vi "未命名 5.vi"(0 "Image In":T3, 1 "Image Dst":T3, 2 "ROI Descriptor (Pattern Matching 1)":T2={"Global Rectangle"=[20, 78, 890, 919], "Contours"=[{"ID"=enum."External", "Type"=12, "Coordinates"=[20, 78, 890, 919, 0]}]} {"Contours"."Type" items=["No Selection", "Point", "Line", "Rectangle", "Oval", "Polygon", "Freehand Region", "Annulus", "Unused2", "Unused3", "Broken Line", "Freehand Line", "Rotated Rectangle"]}, 3 "Algorithm (Pattern Matching 1)":i32(ring)=2 items=["All", "Low Discrepancy Sampling", "Grayscale Value Pyramid", "Gradients Pyramid"], 4 "Parameters (Pattern Matching 1)":T1={"Number of Matches Requested"=1, "Minimum Match Score"=800.0, "Angle Ranges"=[]}, 5 "Advanced Options (Pattern Matching 1)":cluster{"Item":u16, "Value":dbl}[](array[cluster])=[{"Item"=102, "Value"=10.0}, {"Item"=106, "Value"=300.0}, {"Item"=107, "Value"=0.0}, {"Item"=108, "Value"=6.0}, {"Item"=109, "Value"=1.0}, {"Item"=114, "Value"=25.0}, {"Item"=111, "Value"=20.0}, {"Item"=112, "Value"=10.0}, {"Item"=113, "Value"=20.0}, {"Item"=103, "Value"=1.0}, {"Item"=104, "Value"=20.0}, {"Item"=105, "Value"=0.0}, {"Item"=100, "Value"=6.0}] {"Item" items=["LD Sampling - Minimum Constrast"=0, "LD Sampling - Enable Subpixel Accuracy"=1, "LD Sampling - Search Strategy"=2, "LD Sampling - Subpixel Iterations"=3, "LD Sampling - Subpixel Tolerance"=4, "LD Sampling - Initial Match List Length"=5, "LD Sampling - Match List Reduction Factor"=6, "LD Sampling - Initial Step Size"=7, "LD Sampling - Intermediate Angular Accuracy"=8, "-"=9, "Pyramid - Max Pyramid Level"=100, "Pyramid - Minimum Contrast"=102, "Pyramid - Enable Subpixel Accuracy"=103, "Pyramid - Subpixel Iterations"=104, "Pyramid - Subpixel Tolerance"=105, "Pyramid - Initial Match List Length"=106, "Pyramid - Match List Reduction Factor"=107, "Pyramid - Intermediate Angular Accuracy"=108, "Pyramid - Process Border Matches"=109, "Pyramid - Min Match Separation Distance"=111, "Pyramid - Min Match Separation Angle"=112, "Pyramid - Max Match Overlap"=113, "Pyramid - Max Cache in MB"=114, "Pyramid - Clear Cache"=115, "-"=116, "Enable Defect Map"=200]}, 6 "Template File Path (Pattern Matching 1)":path=path "D:/Inspect System/Source Code/Template Program/字符检测定位模板.png", 7 "error in":errorcluster) -> (20 "Image Out":T3, 21 "Matches (Pattern Matching 1)":T4(array[cluster]) {"Bounding Box"."y" format="%.2f"; "Bounding Box"."x" format="%.2f"; "Position"."y" format="%.2f"; "Position"."x" format="%.2f"; "Score" format="%.2f"; "Scale" format="%.2f"; "Angle" format="%.2f"}, 22 "Calibrated Matches (Pattern Matching 1)":T4(array[cluster]) {"Bounding Box"."y" format="%.2f"; "Bounding Box"."x" format="%.2f"; "Position"."y" format="%.2f"; "Position"."x" format="%.2f"; "Score" format="%.2f"; "Scale" format="%.2f"; "Angle" format="%.2f"}, 23 "Number of Matches (Pattern Matching 1)":i32, 27 "error out":errorcluster)   [LabVIEW 2017]
doc: "Creates, edits, and runs vision algorithms using NI Vision Assistant.\n\nWhen you place this Express VI on the block diagram, NI Vision Assistant launches. Create an algorithm using the Vision Assistant processing functions. After you create an algorithm, you can select the controls and indicators that you want to be able to programmatically set in LabVIEW. Double-click the Vision Assistant Express VI to edit the algorithm."
uses:
  <vilib>/vision/Image Controls.llb/IMAQ Image.ctl
  <vilib>/vision/Pattern Matching.llb/IMAQ Curve Parameters.ctl
  <vilib>/vision/Pattern Matching.llb/IMAQ Match Range Setting.ctl
  <vilib>/vision/NI_Vision_Development_Module.lvlib
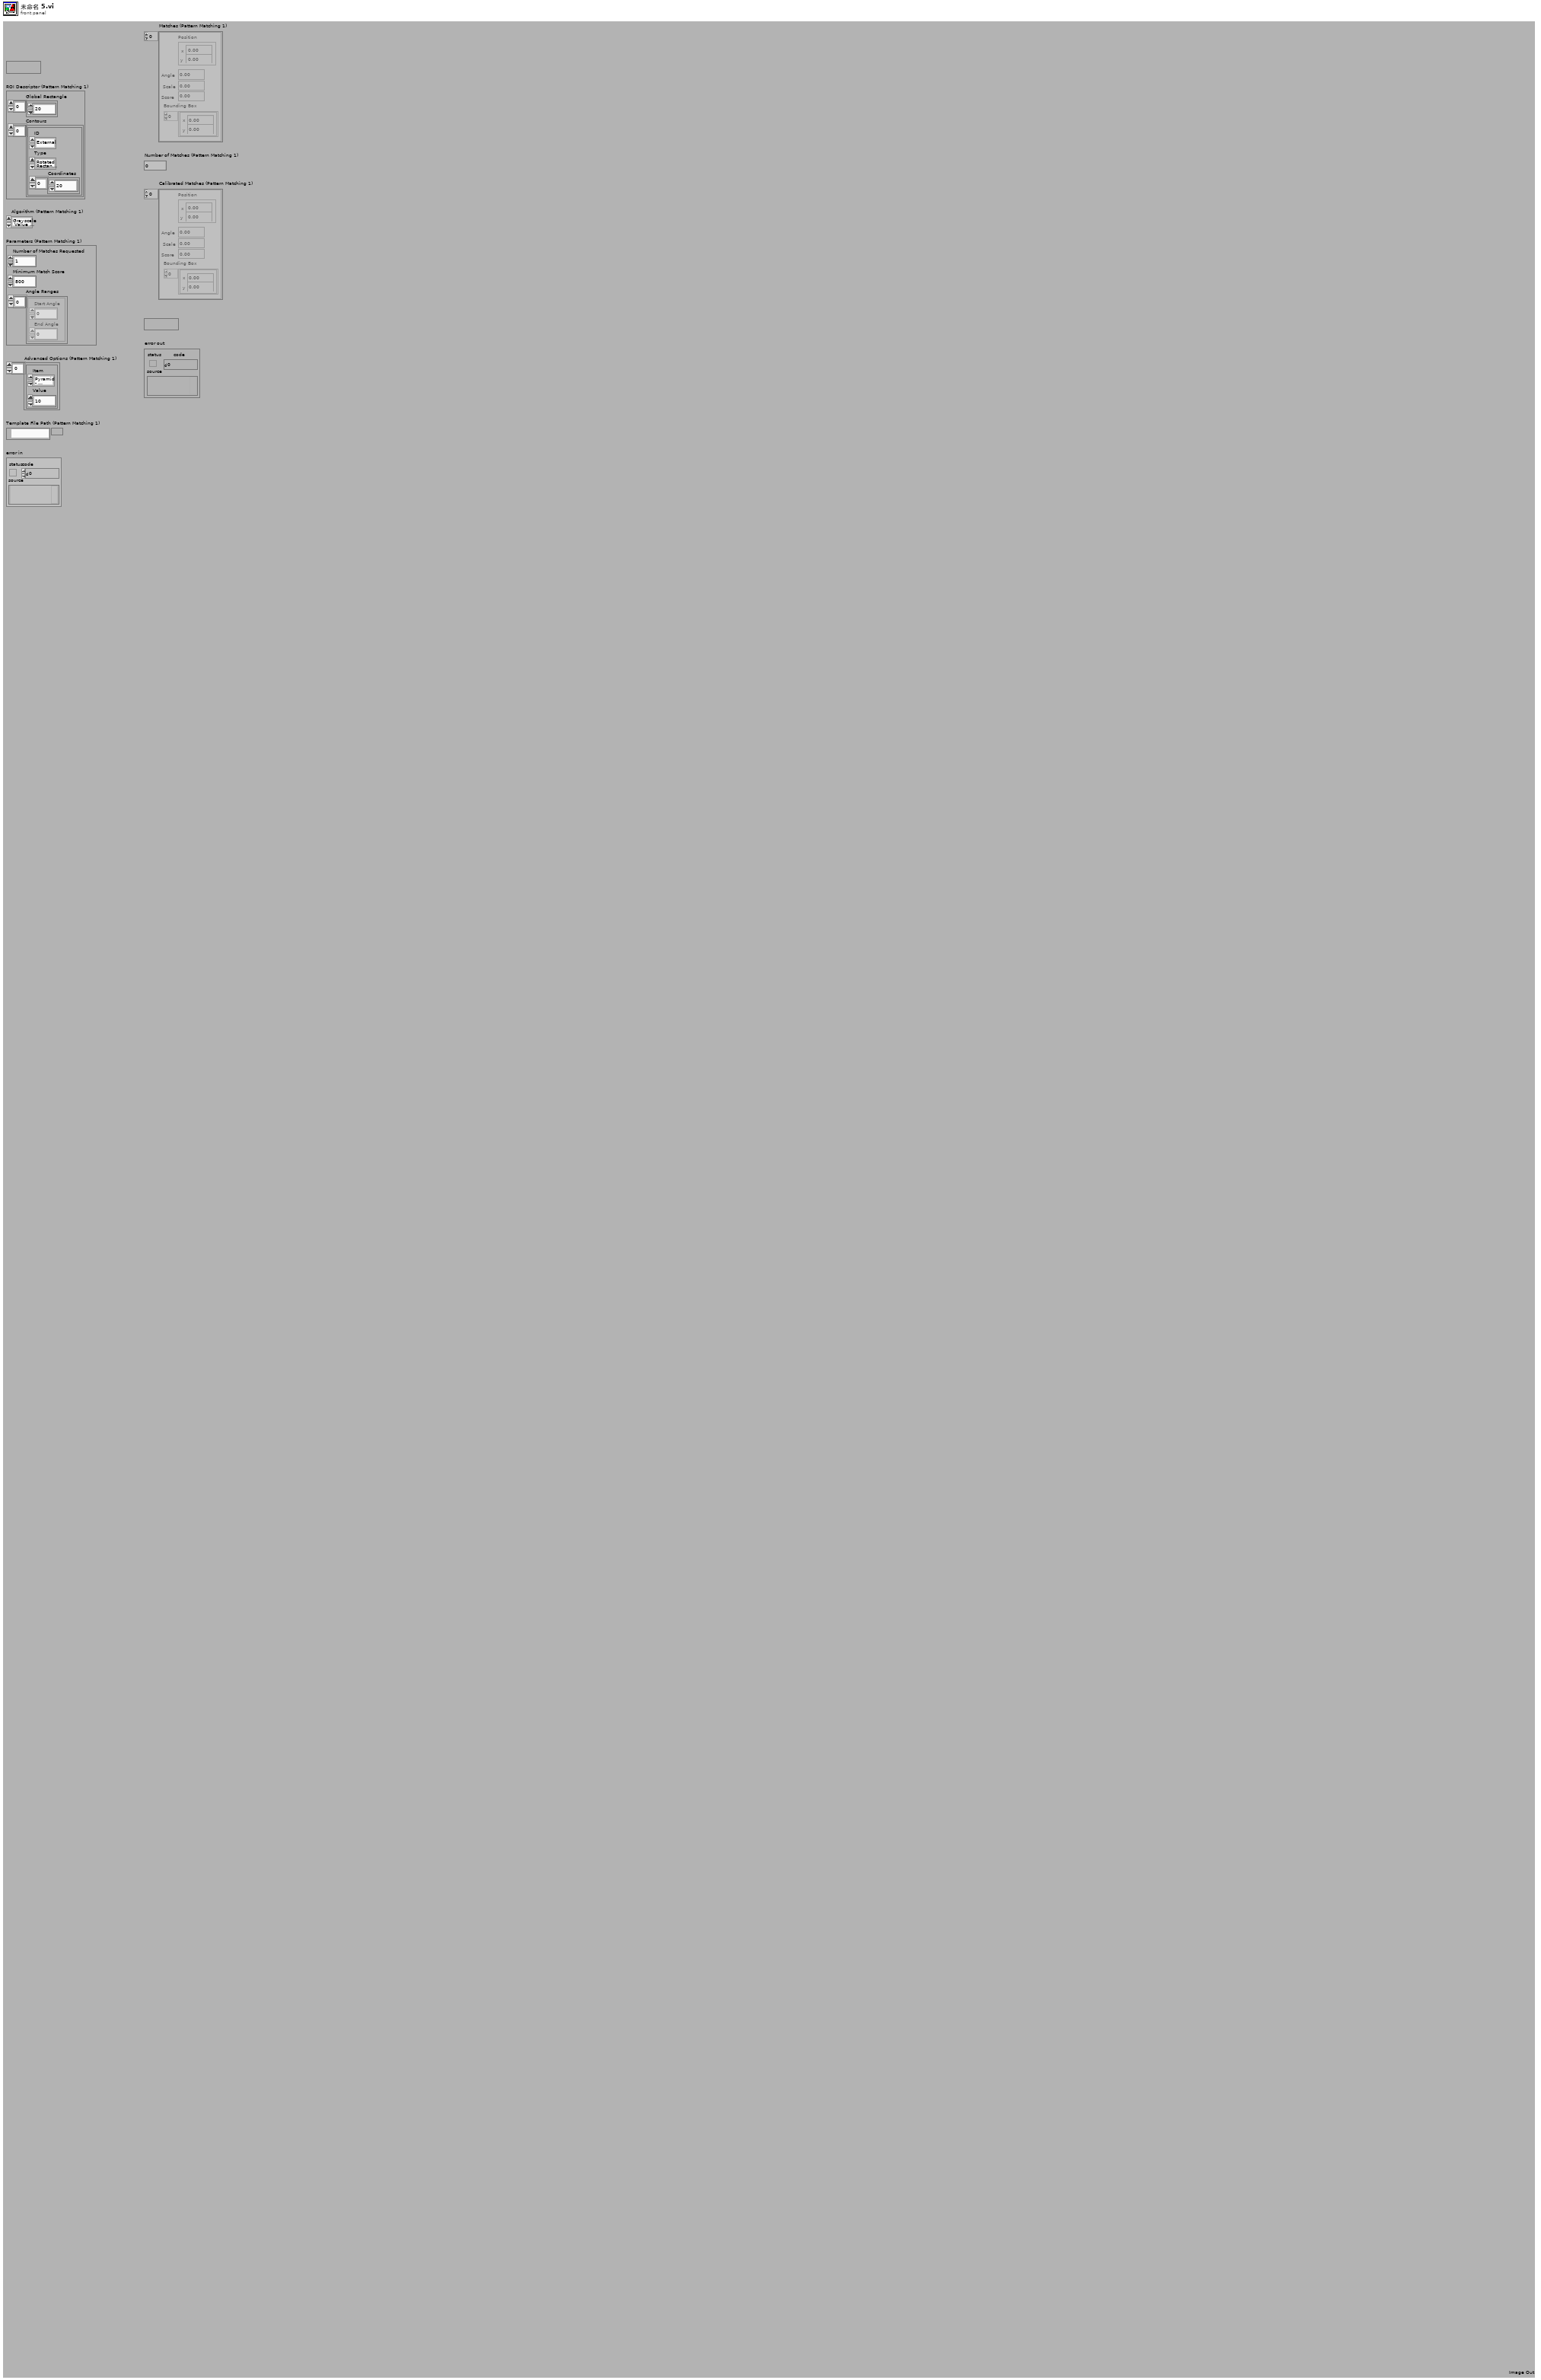
[diagram p1: front panel]
types:
  T1 = cluster{"Number of Matches Requested":i32, "Minimum Match Score":sgl, "Angle Ranges":cluster{"Start Angle":sgl, "End Angle":sgl}[]}
  T2 = cluster{"Global Rectangle":i32[], "Contours":cluster{"ID":enum32{"External", "Internal"}, "Type":u32, "Coordinates":i32[]}[]}
  T3 = typedef "IMAQ Image.ctl" = refnum<image>
  T4 = cluster{"Position":cluster{"x":sgl, "y":sgl}, "Angle":sgl, "Scale":sgl, "Score":sgl, "Bounding Box":cluster{"x":sgl, "y":sgl}[]}[]
  T5 = enum16{"Reset", "Update Coordinate System", "Get Coordinate System"}
  T6 = enum16{"Horizontal Motion", "Vertical Motion", "Horizontal and Vertical Motion", "Horizontal, Vertical and Angular Motion"}
  T7 = cluster{"Origin":cluster{"X":sgl, "Y":sgl}, "Angle (deg)":sgl, "Axis Reference":u32}
  T8 = typedef "IMAQ Curve Parameters.ctl" = cluster{"Extraction Mode":u32, "Edge Threshold":i32, "Edge Filter Size":u32, "Min Length":i32, "Row Search Step Size":i32, "Col Search Step Size":i32, "Max Endpoint Gap":i32, "Closed":bool, "Subpixel":bool}
  T9 = typedef "IMAQ Match Range Setting.ctl" = cluster{"Match Constraints":u32, "Min":dbl, "Max":dbl}
  T10 = cluster{"Curve Parameters":T8, "Match Mode":cluster{"Rotation":bool, "Scale":bool, "Occlusion":bool, "Reserved 1":bool, "Reserved 2":bool, "Reserved 3":bool}, "Range Settings":T9[], "Number of Matches":i32, "Minimum Match Score":sgl, "SubPixel Accuracy":bool, "Adv. Geometric Match Options 2":cluster{"Setup Data Item":u16, "Item Value":dbl}[]}
  T11 = typedef "Image Type" = u32
  T12 = typedef "IMAQ GM Match Report.ctl" = cluster{"Position":cluster{"x":sgl, "y":sgl}, "Angle":sgl, "Scale":sgl, "Score":sgl, "Bounding Box":cluster{"x":sgl, "y":sgl}[], "Contrast Reversed":bool, "Occlusion %":sgl, "Template Target Curve Score":sgl, "Target Template Curve Score":sgl, "Correlation Score":sgl}
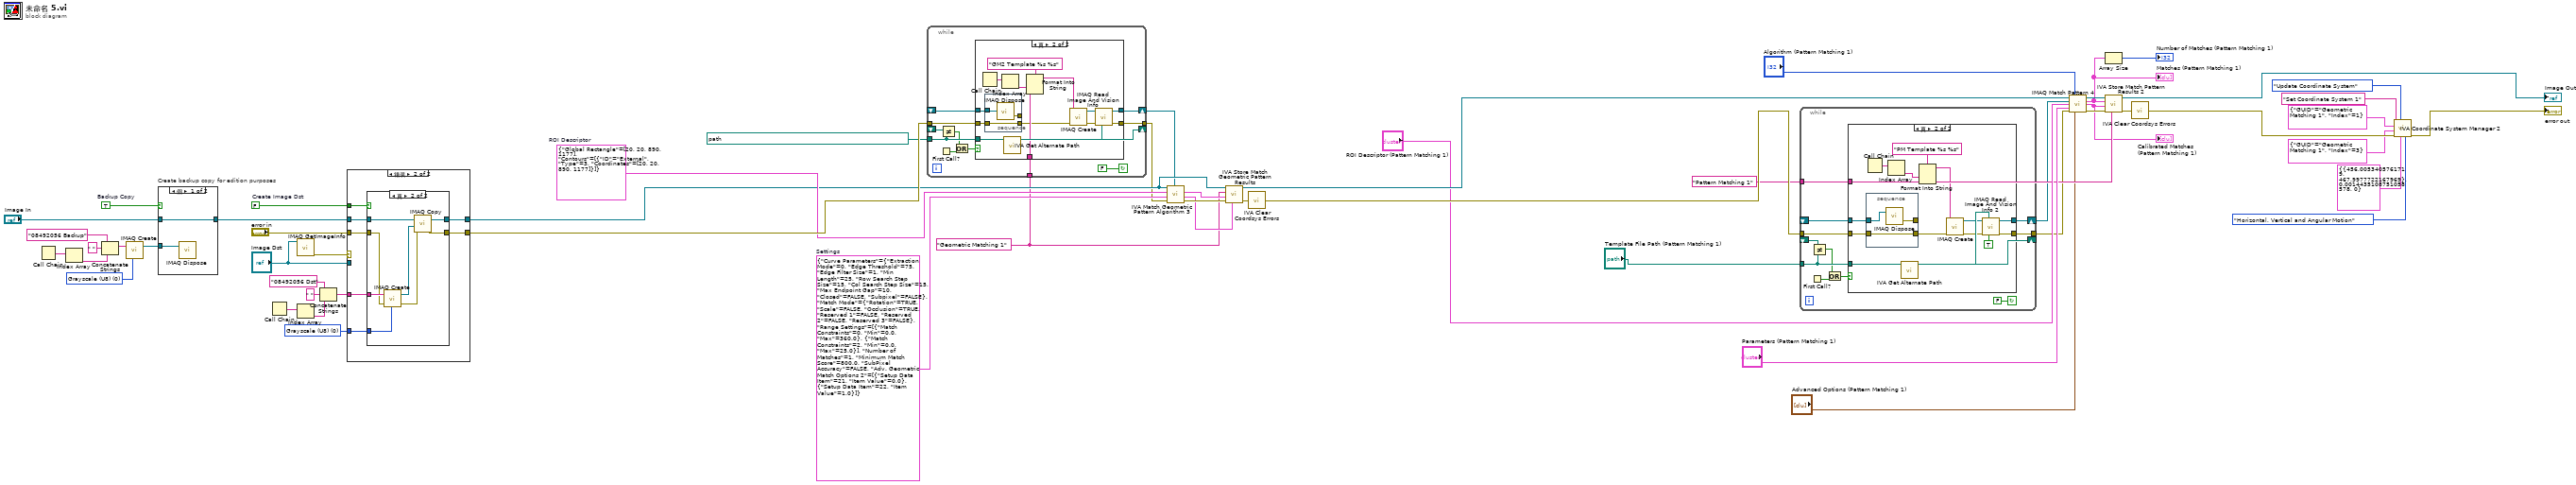
[diagram p0: block diagram]
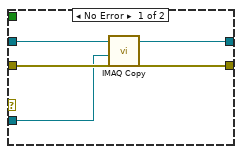
[diagram p4: hidden frame]
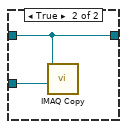
[diagram p6: hidden frame]
diagram:
  w16 = "Pattern Matching 1" ("Step Name")
  w30 = T10 {"Curve Parameters"={"Extraction Mode"=0, "Edge Threshold"=75, "Edge Filter Size"=1, "Min Length"=25, "Row Search Step Size"=15, "Col Search Step Size"=15, "Max Endpoint Gap"=10, "Closed"=FALSE, "Subpixel"=FALSE}, "Match Mode"={"Rotation"=TRUE, "Scale"=FALSE, "Occlusion"=TRUE, "Reserved 1"=FALSE, "Reserved 2"=FALSE, "Reserved 3"=FALSE}, "Range Settings"=[{"Match Constraints"=0, "Min"=0.0, "Max"=360.0}, {"Match Constraints"=2, "Min"=0.0, "Max"=25.0}], "Number of Matches"=1, "Minimum Match Score"=800.0, "SubPixel Accuracy"=FALSE, "Adv. Geometric Match Options 2"=[{"Setup Data Item"=21, "Item Value"=0.0}, {"Setup Data Item"=22, "Item Value"=1.0}]}  # Settings
  w29 = "Geometric Matching 1" ("Step Name")
  w35 = T2 {"Global Rectangle"=[20, 20, 890, 1177], "Contours"=[{"ID"=enum."External", "Type"=3, "Coordinates"=[20, 20, 890, 1177]}]}  # ROI Descriptor
  w37 = T11 0 items=["Grayscale (U8)", "Grayscale (I16)", "Grayscale (SGL)", "Complex (CSG)", "RGB (U32)", "HSL (U32)", "RGB (U64)", "Grayscale (U16)"] ("Image Dst Type")
  w38 = T11 0 items=["Grayscale (U8)", "Grayscale (I16)", "Grayscale (SGL)", "Complex (CSG)", "RGB (U32)", "HSL (U32)", "RGB (U64)", "Grayscale (U16)"] ("Image Type")
  w57 = TRUE  # Backup Copy
  w50 = FALSE  # Create Image Dst
  n1 = Call Chain() -> (call chain=w44:string[])
  n2 = Index Array(array=w44) -> (element=w43:string)  [unwired: 1 in]
  n3 = Concatenate Strings("08492056 Backup" ("Backup Image Name"), " ", w43) -> (w40:string)
  n4 = call "IMAQ Create"("Image Name"=w40, "Image Type"=w38) -> ("New Image"=w39:T3)  [unwired: 2 in, 2 out]
  n5 = case "Create backup copy for edition purposes" shown="假" w57 {
    tunnel: [w59 w61] -> w53
    tunnel: "Image In" -> [w59 w61]
    tunnel: w39 -> [w58 w60]
    frame False {
      n6 = call "IMAQ Dispose"("Image"=w58) -> ()  [unwired: 2 in, 4 out]
    }
    frame True {
      n7 = call "IMAQ Copy"("Image Dst"=w60, "Image Src"=w61) -> ()  [unwired: 1 in, 5 out]
    }
  }
  n8 = Call Chain() -> (call chain=w49:string[])
  n9 = call "IMAQ GetImageInfo"("Image"="Image Dst") -> ("error out"=w55:errorcluster)  [unwired: 1 in, 9 out]
  n10 = Index Array(array=w49) -> (element=w47:string)  [unwired: 1 in]
  n11 = Concatenate Strings("08492056 Dst" ("Image Dst Name"), " ", w47) -> (w45:string)
  n12 = case "条件结构" shown="错误" w55 {
    tunnel: [w66 w70] -> w31
    tunnel: [w65 w69] -> w51
    tunnel: w53 -> [w64 w71]
    tunnel: "error in" -> [w63 w67]
    tunnel: "Image Dst" -> [w62 _]
    tunnel: w45 -> [_ w73]
    tunnel: w37 -> [_ w72]
    tunnel: w50 -> [_ w68]
    frame No Error {
      n13 = call "IMAQ Copy"("error in (no error)"=w63, "Image Dst"=w62, "Image Src"=w64) -> ("error out"=w65:errorcluster, "Image Dst Out"=w66:T3)  [unwired: 3 out]
    }
    frame Error {
      n14 = case "条件结构" shown="真" w68 {
        tunnel: w73 -> [_ w83]
        tunnel: w72 -> [_ w82]
        tunnel: w71 -> [w75 w80]
        tunnel: [w75 w79] -> w70
        tunnel: [w74 w78] -> w69
        tunnel: w67 -> [w74 w76]
        frame False {
        }
        frame True {
          n15 = call "IMAQ Create"("Image Name"=w83, "Image Type"=w82, "error in (no error)"=w76) -> ("New Image"=w81:T3, "error out"=w77:errorcluster)  [unwired: 1 in, 1 out]
          n16 = call "IMAQ Copy"("error in (no error)"=w77, "Image Dst"=w81, "Image Src"=w80) -> ("error out"=w78:errorcluster, "Image Dst Out"=w79:T3)  [unwired: 3 out]
        }
      }
    }
  }
  n17 = while {
    shift-right: [w94] -> w27
    shift-left: _ -> [w93]
    tunnel: [w91] -> w28
    tunnel: w51 -> [w90]
    tunnel: path "D:/Inspect System/Source Code/SubVIs/字符检测VI/aaaa.png" ("Template File Path") -> [w87]
    tunnel: w29 -> [w89]
    shift-right: [w87] -> _
    shift-left: _ -> [w88]
    stop <- FALSE continue-if-true
    n18 = First Call?() -> (First Call?: T/F=w86:bool)
    n19 = Not Equal?(x=w88, y=w87) -> (x != y?=w85:bool)
    n20 = Or(x=w85, y=w86) -> (x .or. y?=w84:bool)
    n21 = case "条件结构" shown="真" w84 {
      tunnel: [w96 w108] -> w94
      tunnel: w93 -> [w96 w100]
      tunnel: [w95 w105] -> w91
      tunnel: w90 -> [w95 w101]
      tunnel: w89 -> [_ w102]
      tunnel: w87 -> [_ w99]
      frame False {
      }
      frame True {
        n22 = Call Chain() -> (call chain=w104:string[])
        n23 = stacked-sequence "层叠式顺序结构" {
          tunnel: w101 -> [w113]
          tunnel: w100 -> [w112]
          tunnel: [w113] -> w97
          tunnel: [w111] -> _
          frame #0 {
            n24 = call "IMAQ Dispose"("Image"=w112) -> ("error out"=w111:errorcluster)  [unwired: 2 in, 3 out]
          }
        }
        n25 = Index Array(array=w104) -> (element=w103:string)  [unwired: 1 in]
        n26 = call <vilib>:"IVA Get Alternate Path.vi"("Path In"=w99) -> ("Path Out"=w98:path)  [unwired: 10 out]
        n27 = Format Into String(format string="GM2 Template %s %s" ("Image Name"), w103, w102) -> (resulting string=w110:string)  [unwired: 2 in, 1 out]
        n28 = call "IMAQ Create"("Image Name"=w110, "error in (no error)"=w97) -> ("New Image"=w107:T3, "error out"=w106:errorcluster)  [unwired: 2 in, 1 out]
        n29 = call "IMAQ Read Image And Vision Info"("File Path"=w98, "error in (no error)"=w106, "Image"=w107) -> ("error out"=w105:errorcluster, "Image Out"=w108:T3)  [unwired: 1 in, 6 out]
      }
    }
  }
  n30 = call <vilib>:"IVA Match Geometric Pattern Algorithm 3.vi"("Template"=w27, "error in (no error)"=w28, "Settings"=w30, "ROI Descriptor"=w35, "Image"=w31) -> ("error out"=w34:errorcluster, "Calibrated Matches"=w32:T12[], "Matches"=w33:T12[])  [unwired: 4 out]
  n31 = call <vilib>:"IVA Store Match Geometric Pattern Results.vi"("Calibrated Matches"=w32, "error in (no error)"=w34, "Matches"=w33, "Step Name"=w29, "Image in"=w31) -> ("error out"=w26:errorcluster, "Image dup"=w23:T3)  [unwired: 5 out]
  n32 = call <vilib>:"IVA Clear Coordsys Errors.vi"("error in (no error)"=w26) -> ("error out"=w25:errorcluster)  [unwired: 10 in]
  n33 = while {
    shift-right: [w124] -> w13
    shift-left: _ -> [w123]
    tunnel: [w121] -> w12
    tunnel: w25 -> [w120]
    tunnel: "Template File Path (Pattern Matching 1)" -> [w117]
    tunnel: w16 -> [w119]
    shift-right: [w117] -> _
    shift-left: _ -> [w118]
    stop <- FALSE continue-if-true
    n34 = First Call?() -> (First Call?: T/F=w116:bool)
    n35 = Not Equal?(x=w118, y=w117) -> (x != y?=w115:bool)
    n36 = Or(x=w115, y=w116) -> (x .or. y?=w114:bool)
    n37 = case "条件结构" shown="真" w114 {
      tunnel: [w126 w131] -> w124
      tunnel: w123 -> [w126 w135]
      tunnel: [w125 w132] -> w121
      tunnel: w120 -> [w125 w134]
      tunnel: w117 -> [_ w136]
      tunnel: w119 -> [_ w137]
      frame False {
      }
      frame True {
        n38 = stacked-sequence "层叠式顺序结构" {
          tunnel: w135 -> [w144]
          tunnel: w134 -> [w143]
          tunnel: [w143] -> w128
          tunnel: [w142] -> _
          frame #0 {
            n39 = call "IMAQ Dispose"("Image"=w144) -> ("error out"=w142:errorcluster)  [unwired: 2 in, 3 out]
          }
        }
        n40 = Call Chain() -> (call chain=w139:string[])
        n41 = Index Array(array=w139) -> (element=w138:string)  [unwired: 1 in]
        n42 = call <vilib>:"IVA Get Alternate Path.vi"("Path In"=w136) -> ("Path Out"=w133:path)  [unwired: 10 out]
        n43 = Format Into String(format string="PM Template %s %s" ("Image Name"), w138, w137) -> (resulting string=w141:string)  [unwired: 2 in, 1 out]
        n44 = call "IMAQ Create"("Image Name"=w141, "error in (no error)"=w128) -> ("New Image"=w130:T3, "error out"=w129:errorcluster)  [unwired: 2 in, 1 out]
        n45 = call "IMAQ Read Image And Vision Info 2"("Use File Path Image Type"=TRUE, "File Path"=w133, "error in (no error)"=w129, "Image"=w130) -> ("error out"=w132:errorcluster, "Image Out"=w131:T3)  [unwired: 5 in, 1 out]
      }
    }
  }
  n46 = call "IMAQ Match Pattern 4"("Image"=w23, "Algorithm"="Algorithm (Pattern Matching 1)", "Template Image"=w13, "ROI Descriptor"="ROI Descriptor (Pattern Matching 1)", "Parameters"="Parameters (Pattern Matching 1)", "error in (no error)"=w12, "Advanced Options"="Advanced Options (Pattern Matching 1)") -> ("Image (duplicate)"=w21:T3, "Matches (pixel)"=w15:T4, "Matches (real-world)"=w14:T4, "error out"=w22:errorcluster)  [unwired: 4 in, 1 out]
  "Matches (Pattern Matching 1)" <- w15
  "Calibrated Matches (Pattern Matching 1)" <- w14
  n47 = Array Size(array=w15) -> (size(s)=→"Number of Matches (Pattern Matching 1)":i32)
  n48 = call <vilib>:"IVA Store Match Pattern Results 2.vi"("Step Name"=w16, "error in (no error)"=w22, "Matches (real-world)"=w14, "Matches (pixel)"=w15, "Image in"=w21) -> ("error out"=w11:errorcluster, "Image dup"=→"Image Out":T3)  [unwired: 1 in, 4 out]
  n49 = call <vilib>:"IVA Clear Coordsys Errors.vi"("error in (no error)"=w11) -> ("error out"=w10:errorcluster)  [unwired: 10 in]
  n50 = call <vilib>:"IVA Coordinate System Manager 2.vi"("Mode"=T6."Horizontal, Vertical and Angular Motion", "Reference System"=T7 {"Origin"={"X"=456.00534, "Y"=467.99777}, "Angle (deg)"=0.0014435109, "Axis Reference"=0}, "Function"=T5."Update Coordinate System", "error in (no error)"=w10, "Angle ID"=cluster{"GUID":string, "Index":i32} {"GUID"="Geometric Matching 1", "Index"=3}, "Origin ID"=cluster{"GUID":string, "Index":i32} {"GUID"="Geometric Matching 1", "Index"=1}, "Coordinate System Name"="Set Coordinate System 1") -> ("error out"=→"error out":errorcluster)  [unwired: 4 out]
